vi "TrajectoryConfig_setKinematicsSwerveDrive.vi"(9 "SWERVE_DRIVE_KINEMATICS":T1 {"SavedModuleStates"."Angle"."SIN" format="%13.4f"; "SavedModuleStates"."Angle"."COS" format="%13.4f"; "SavedModuleStates"."Angle"."VALUE" format="%13.4f"; "PrevCoR"."Y" format="%14.3f"; "PrevCoR"."X" format="%14.3f"; "Modules"."Y" format="%14.3f"; "Modules"."X" format="%14.3f"}, 11 "inTRAJECTORY_CONFIG":T6 {"End Velocity" format="%20.4f"; "StartVelocity" format="%20.4f"; "Max Acceleration" format="%20.4f"; "MaxVelocity" format="%20.4f"}) -> (3 "outTRAJECTORY_CONFIG":T6 {"End Velocity" format="%20.4f"; "StartVelocity" format="%20.4f"; "Max Acceleration" format="%20.4f"; "MaxVelocity" format="%20.4f"})   [LabVIEW 2019, in "Trajectory_Library.lvlib"]
doc: "Adds and enabled a swerve drive kinematics constraint to ensure that no wheel velocity of a swerve drive goes above the max velocity. The TrajectoryConfiguration max velocity is used for the swerve drive max individual wheel velocity.\n\nParameters:\n - SwerveDriveKinematics - The swerve drive kinematics data structure\n - InTrajectoryConfig - The trajectory configuration data structure\n\nReturns:\n - OutTrajectoryConfig - Modified trajectory configuration data structure"
uses:
  Trajectory_Library.lvlib
  TypeDef/TRAJ_CONFIG.ctl
  <vilib>/Analysis/Matrix/Datatypes/RealMatrix.ctl
  <vilib>/Analysis/Matrix/NI_Matrix.lvlib
  TypeDef/TRANSLATION2D.ctl
  TypeDef/SWERVE_DRIVE_KINEMATICS.ctl
  TypeDef/ROTATION2D.ctl
  TypeDef/SWERVE_DRIVE_MODULE_STATE.ctl
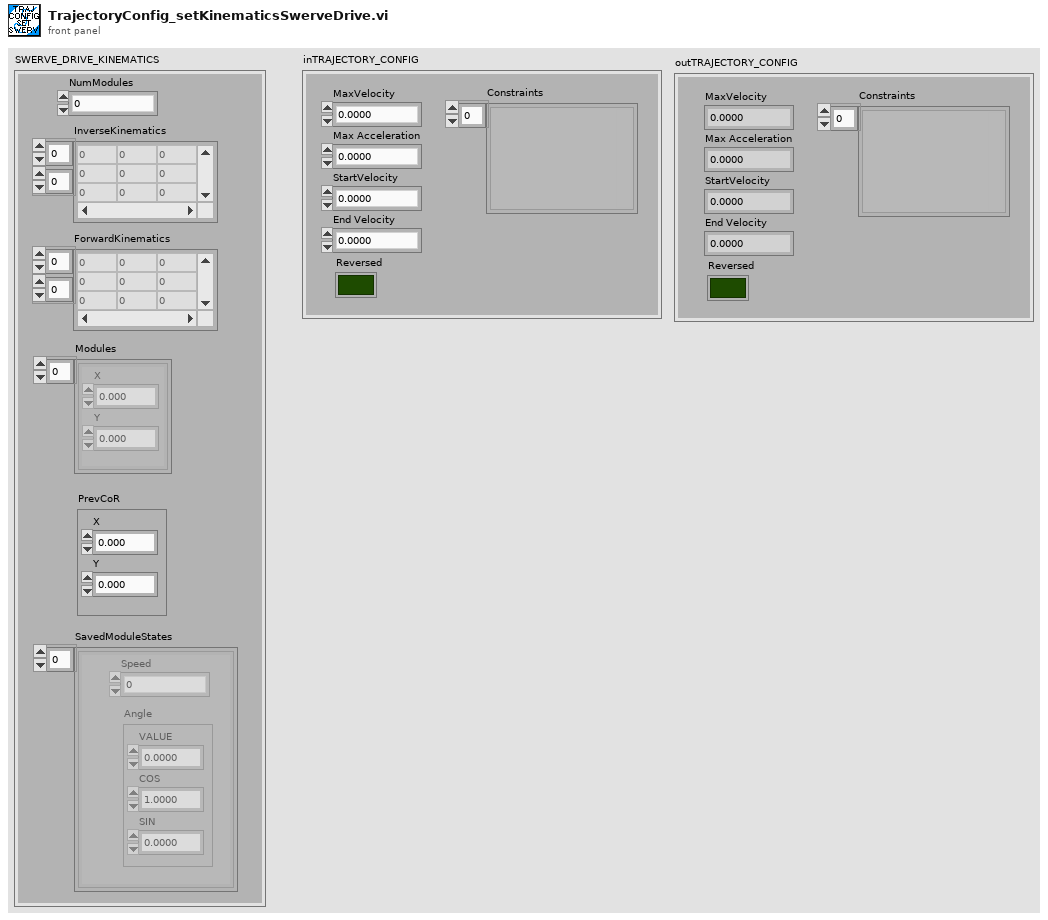
[diagram p1: front panel]
types:
  T1 = typedef "Trajectory_Library.lvlib/SWERVE_DRIVE_KINEMATICS.ctl" = cluster{"NumModules":i32, "InverseKinematics":T2, "ForwardKinematics":T2, "Modules":T3[], "PrevCoR":T3, "SavedModuleStates":T4[]}
  T2 = typedef "NI_Matrix.lvlib/RealMatrix.ctl" = dbl[][]
  T3 = typedef "Trajectory_Library.lvlib/TRANSLATION2D.ctl" = cluster{"X":dbl, "Y":dbl}
  T4 = typedef "Trajectory_Library.lvlib/SWERVE_DRIVE_MODULE_STATE.ctl" = cluster{"Speed":dbl, "Angle":T5}
  T5 = typedef "Trajectory_Library.lvlib/ROTATION2D.ctl" = cluster{"VALUE":dbl, "COS":dbl, "SIN":dbl}
  T6 = typedef "Trajectory_Library.lvlib/TRAJ_CONFIG.ctl" = cluster{"MaxVelocity":dbl, "Max Acceleration":dbl, "StartVelocity":dbl, "End Velocity":dbl, "Reversed":bool, "Constraints":variant[]}
  T7 = typedef "WPILib_Math.lvlib/TRAJ_CONSTRAINT_SWERVE_DRIVE_KINEMATICS.ctl" = cluster{"Max Speed (M/S)":dbl, "SwerveKinematics":T8}
  T8 = typedef "WPILib_Math.lvlib/SWERVE_DRIVE_KINEMATICS.ctl" = cluster{"NumModules":i32, "InverseKinematics":T2, "ForwardKinematics":T2, "Modules":T9[], "PrevCoR":T9, "SavedModuleStates":T10[]}
  T9 = typedef "WPILib_Math.lvlib/TRANSLATION2D.ctl" = cluster{"X":dbl, "Y":dbl}
  T10 = typedef "WPILib_Math.lvlib/SWERVE_DRIVE_MODULE_STATE.ctl" = cluster{"Speed":dbl, "Angle":T11}
  T11 = typedef "WPILib_Math.lvlib/ROTATION2D.ctl" = cluster{"VALUE":dbl, "COS":dbl, "SIN":dbl}
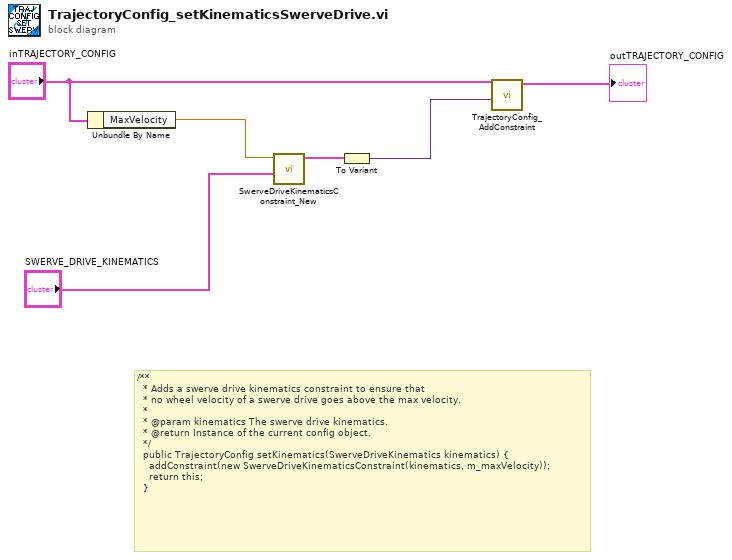
[diagram p0: block diagram]
diagram:
  # "/**\n  * Adds a swerve drive kinematics constraint to ensure that\n  * no wheel velocity of a swerve drive goes above the max velocity.\n  *\n  * @param kinematics The swerve drive kinematics.\n  * @return Instance of the current config object.\n  */\n  public TrajectoryConfig setKinematics(SwerveDriveKinematics kinematics) {\n    addConstraint(new SwerveDriveKinematicsConstraint(kinematics, m_maxVelocity));\n    return this;\n  }"
  n1 = Unbundle By Name("inTRAJECTORY_CONFIG") -> ("MaxVelocity"=w6:dbl)
  n2 = call "SwerveDriveKinematicsConstraint_New.vi"("SwerveKinematics"="SWERVE_DRIVE_KINEMATICS", "Max Speed (M/S)"=w6) -> ("SWERVE_DRIVE_KINE_CONSTRAINT"=w1:T7)  [unwired: 9 in]
  n3 = To Variant(anything=w1) -> (Variant=w4:variant)
  n4 = call "TrajectoryConfig_AddConstraint.vi"("Constraint"=w4, "inTRAJECTORY_CONFIG"="inTRAJECTORY_CONFIG") -> ("outTRAJECTORY_CONFIG"=→"outTRAJECTORY_CONFIG":T6)  [unwired: 9 in]
